vi "Path_Check if File or Folder Exists.vi"(11 "File or Folder Path in":path) -> (2 "File or Folder Found?":bool, 3 "File or Folder Path dub":path)   [LabVIEW 2019, in "ClassLoader.lvlib"]
doc: "Check if a file or folder exists at the given path."
uses:
  ClassLoader.lvlib
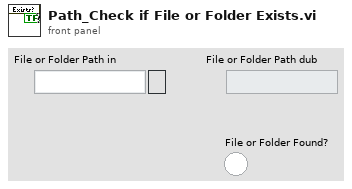
[diagram p1: front panel]
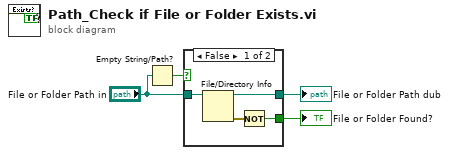
[diagram p0: block diagram]
diagram:
  n1 = Empty String/Path?(string/path="File or Folder Path in") -> (empty?=w1:bool)
  n2 = case shown="False" w1 {
    tunnel: [w8 w9] -> w4
    tunnel: [w6 _] -> w3
    tunnel: "File or Folder Path in" -> [w5 w9]
    frame False {
      n3 = File/Directory Info(path=w5) -> (path out=w8:path, error out=w7:errorcluster)  [unwired: 1 in, 5 out]
      n4 = Not(x=w7) -> (.not. x?=w6:bool)
    }
    frame True {
    }
  }
  "File or Folder Found?" <- w3
  "File or Folder Path dub" <- w4
